vi "Nimbelink_Database_Ops.vi"(0 "Operation":T1(ring)=enum."Get Col Names", 1 "Record data":string[](array[string])=["wo12345", "123450001", "70B3D55A8100", "A1001234567890", "Joe", "2013-05-07 10:28:19", "100013", "353123456789012", "89123456789012345678", "612-555-1212", "Pass", "", "", "", "", "", "", "", "", "", "", "", "", "", "", "", "", "", "", "", "", "", "", "", "", "", "", "", "", "", "", "", "", "", "", "", "", "", "", "", "", "", "", "", "", "", "", "", "", "", "", "", "12:01:00"], 2 "Open SQL session?":bool=TRUE, 3 "Connection In":refnum<k7>, 4 "SQL Query":string="Insert into dbo.test_data VALUES ", 5 "Error in (no error)":errorcluster, 6 "Find column":u16(ring) items=["work_order", "btw_sn", "mac", "meid", "operator", "datetime", "part_number", "imei", "sim_id", "phone", "test_result"], 7 "Find data":string, 10 "table name":string="test_data", 11 "Insert fields":i32=23) -> (12 "Found?":bool, 13 "Last test passed?":bool, 14 "RecordSet":string[][](array[string]), 15 "Column Names":string[](array[string])=["work_order", "btw_sn", "mac", "meid", "operator", "date_time", "part_number", "imei", "sim_id", "phone_number", "test_result", "board_sn", "test_time", "test_program", "test_version", "extra1", "extra2", "guid", "extra3", "extra4", "extra5", "extra6", "extra7"], 16 "Connection Out":refnum<k7>, 17 "Find return string":string, 18 "Records":i32, 19 "Error out":errorcluster)   [LabVIEW 2013]
panel:
  out "Final query string":string="select column_name,* from information_schema.columns\n where table_name = 'test_data'\norder by ordinal_position"
  in  "ConnectionString":string="Provider=SQLOLEDB.1;User Id=SSTest;Password=test;Initial Catalog=Nimbelink;Data Source=BTWSQLSVR\\TESTDEPT "
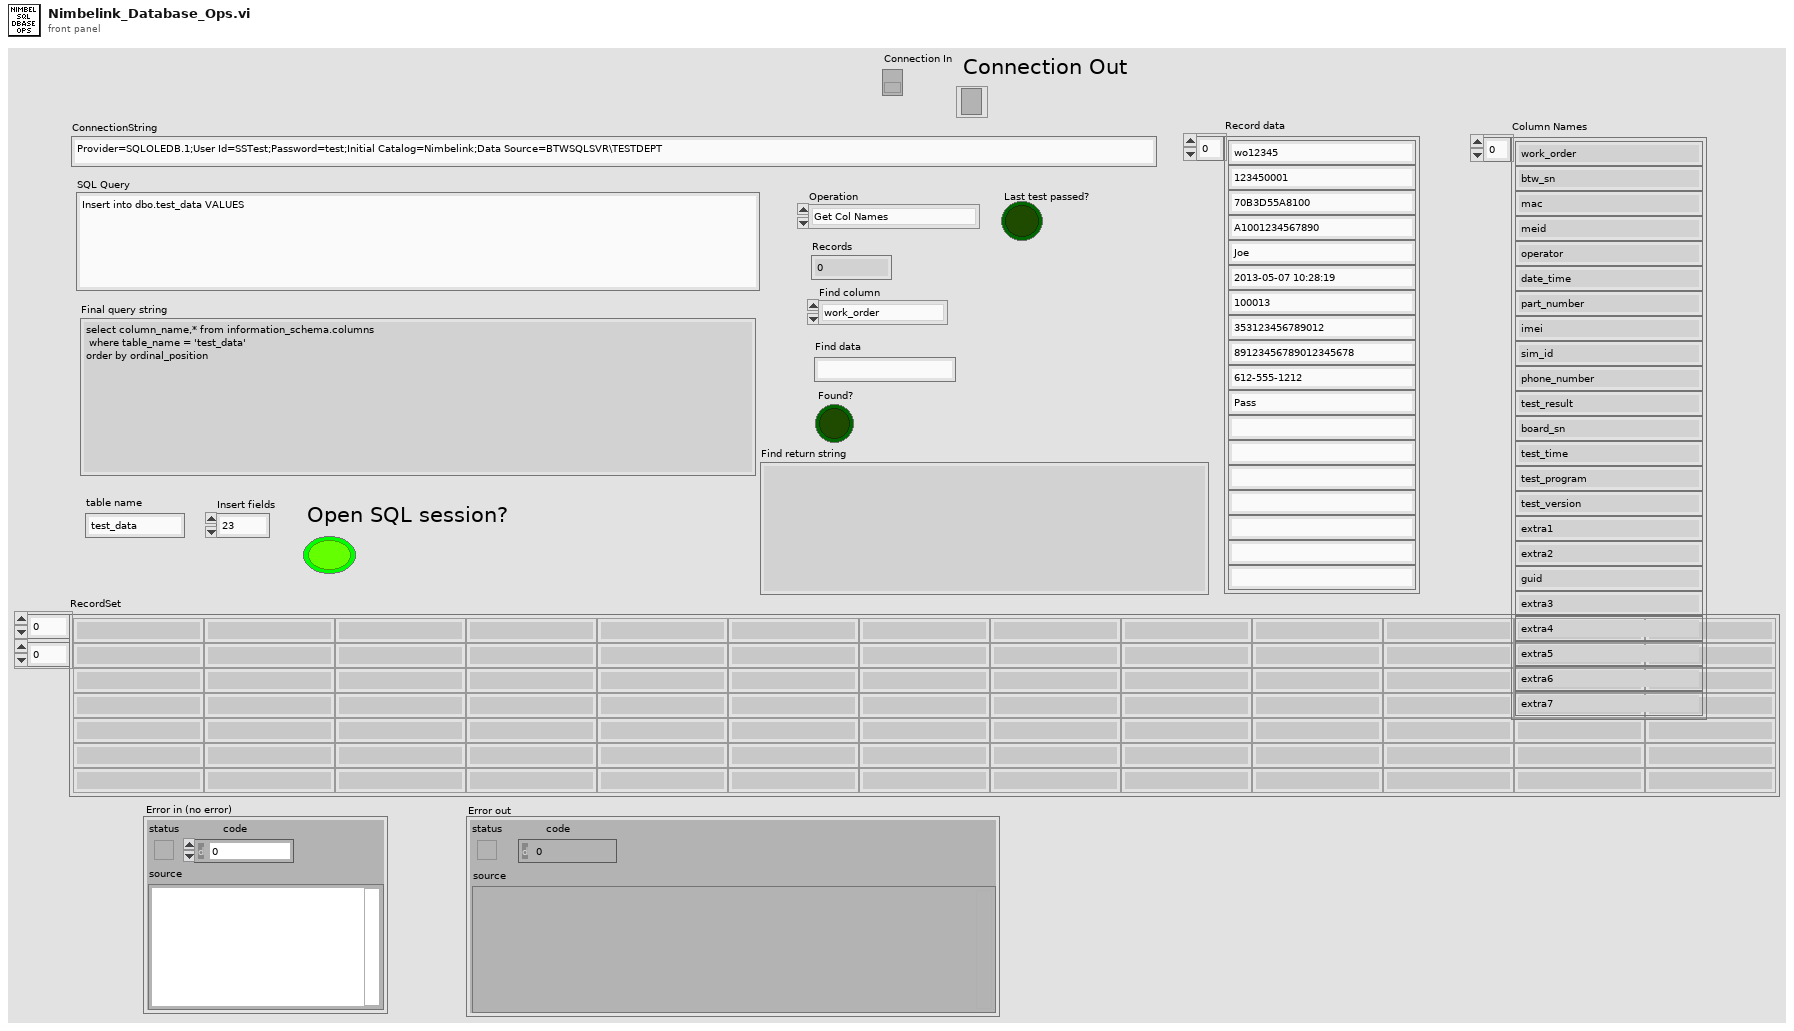
[diagram p1: front panel]
types:
  T1 = enum16{"Query", "Insert", "Select", "Dump Recs", "Get Rec Count", "Get Col Names", "Insert all fields", "Find", "Get last test result", "Get work order qty", "Set work order qty", "Save test report", "Get test report", "Execute query no data", "Select count", "Query and return row 0 col 0"}
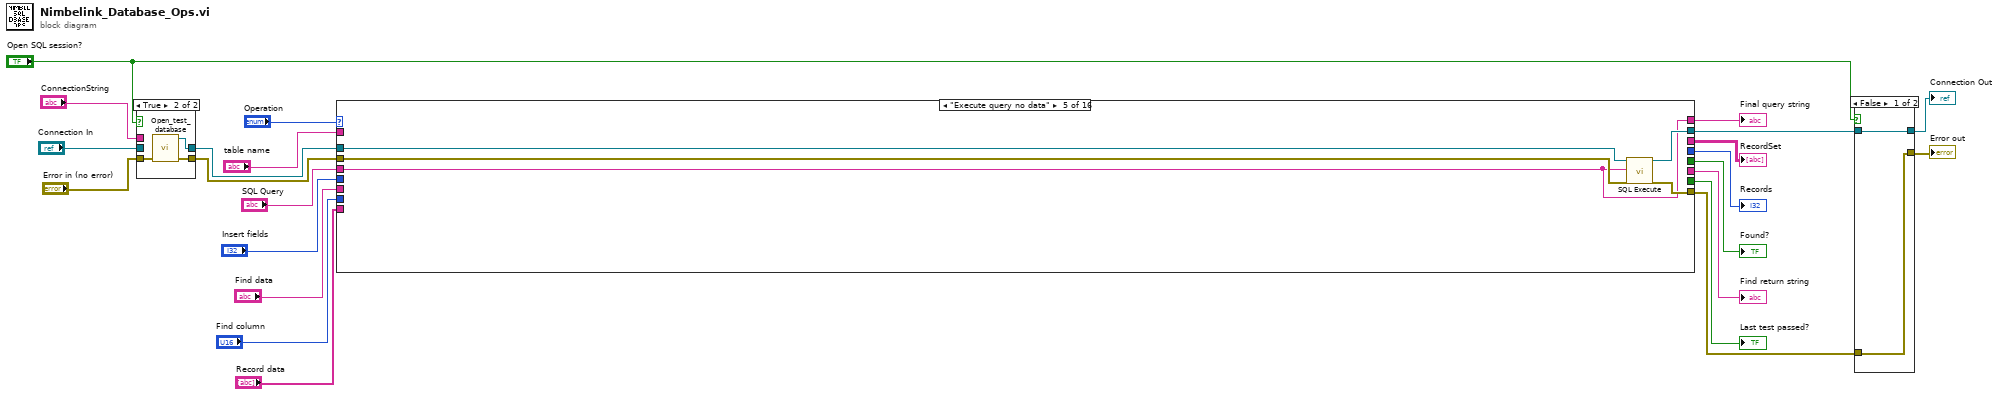
[diagram p0: block diagram]
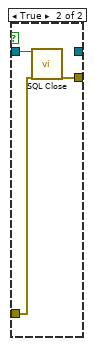
[diagram p2: hidden frame]
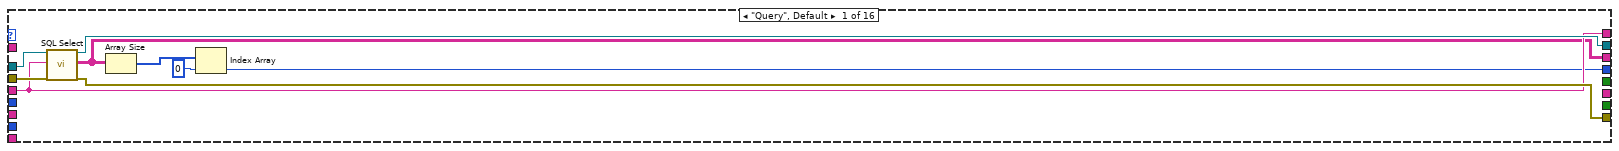
[diagram p4: hidden frame]
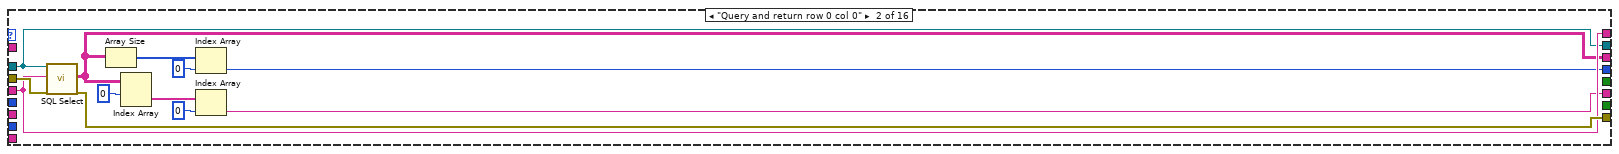
[diagram p5: hidden frame]
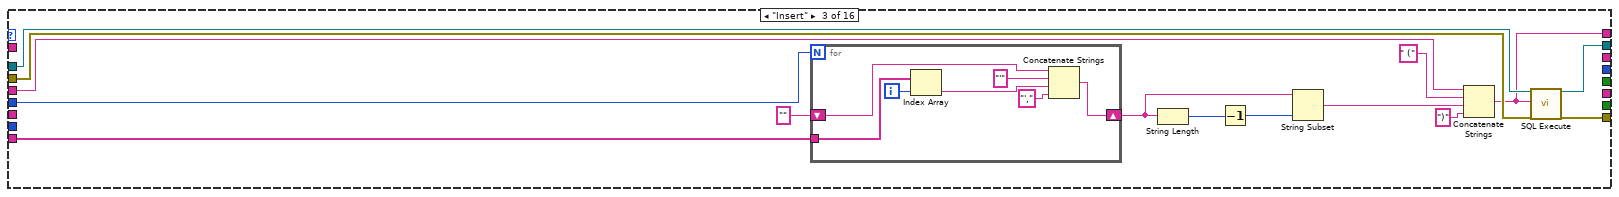
[diagram p6: hidden frame]
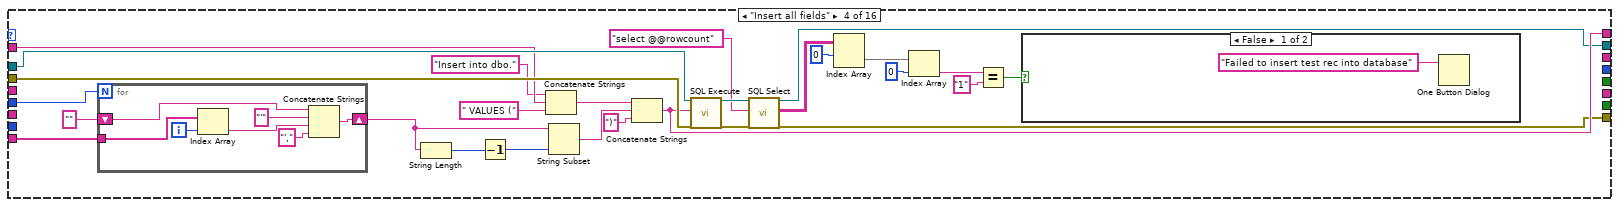
[diagram p7: hidden frame]
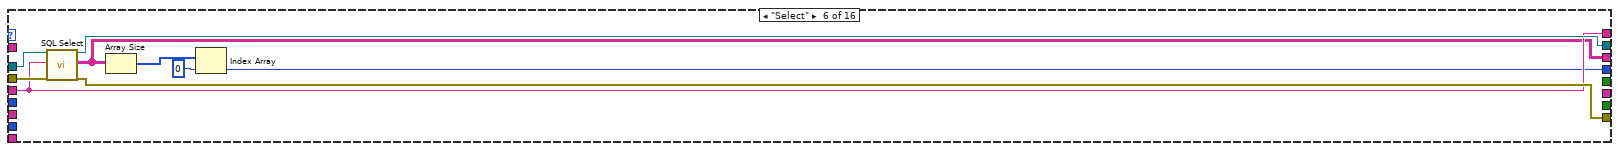
[diagram p9: hidden frame]
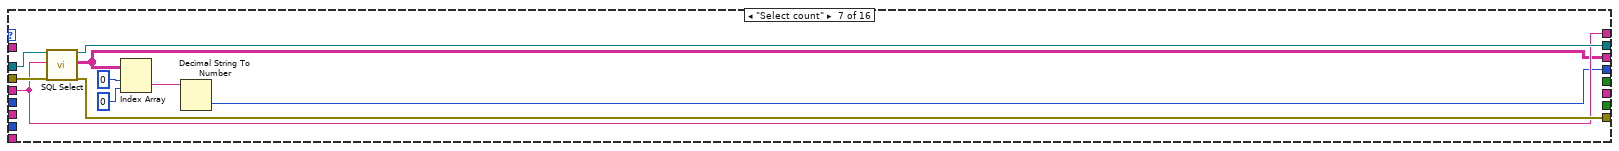
[diagram p10: hidden frame]
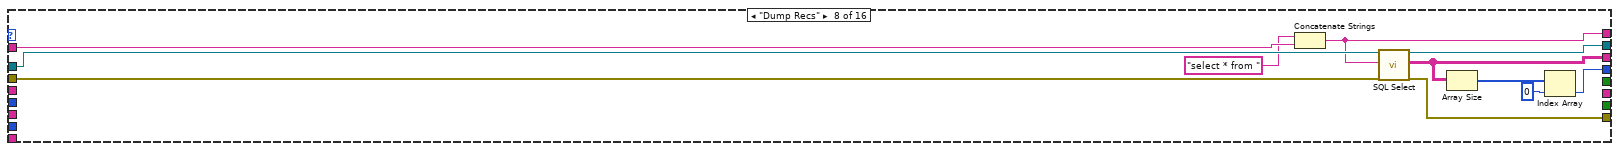
[diagram p11: hidden frame]
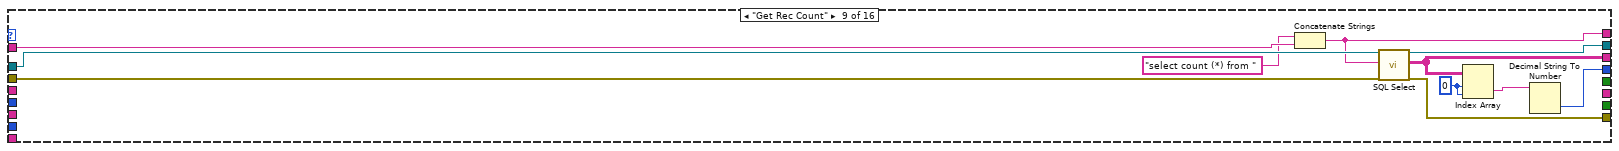
[diagram p12: hidden frame]
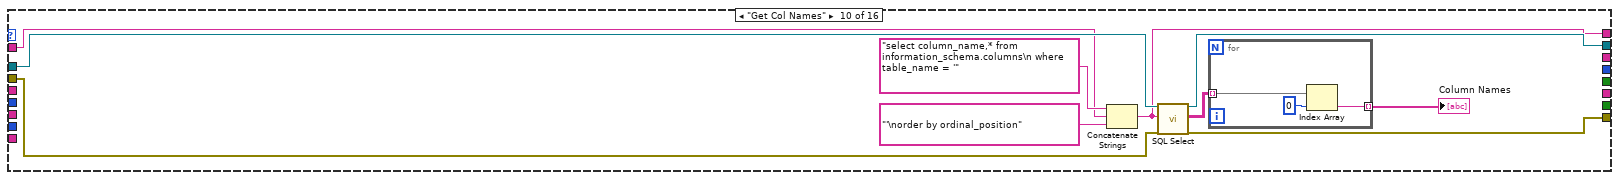
[diagram p13: hidden frame]
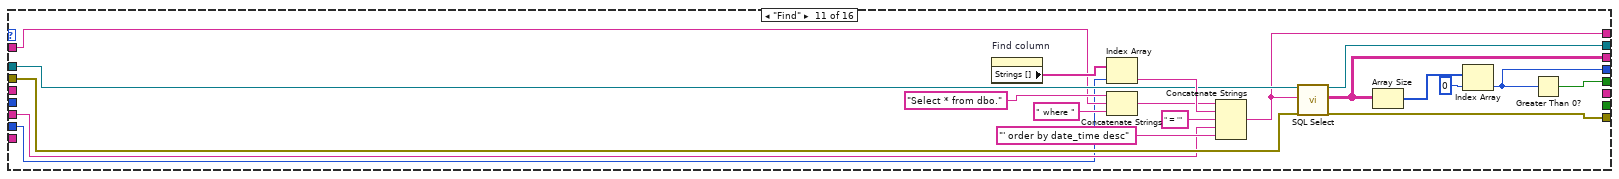
[diagram p14: hidden frame]
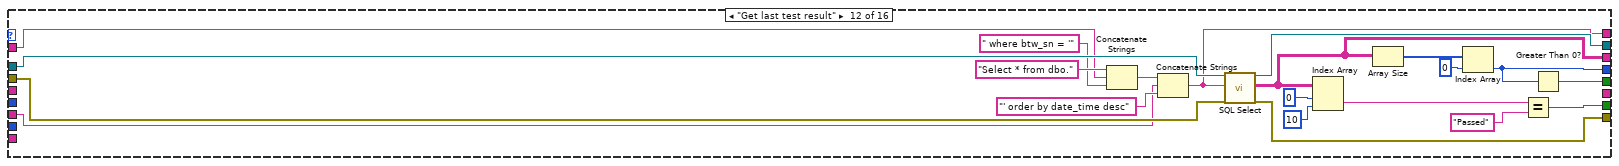
[diagram p15: hidden frame]
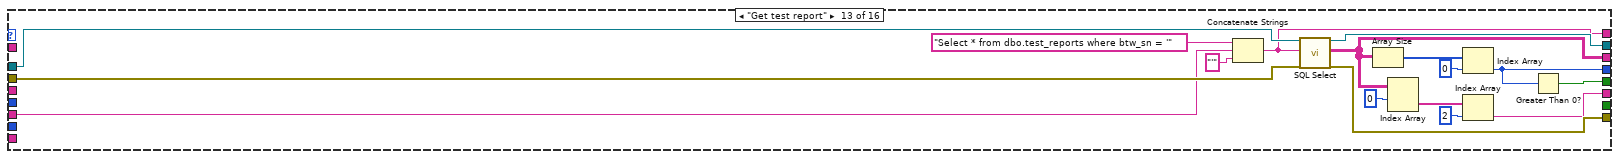
[diagram p16: hidden frame]
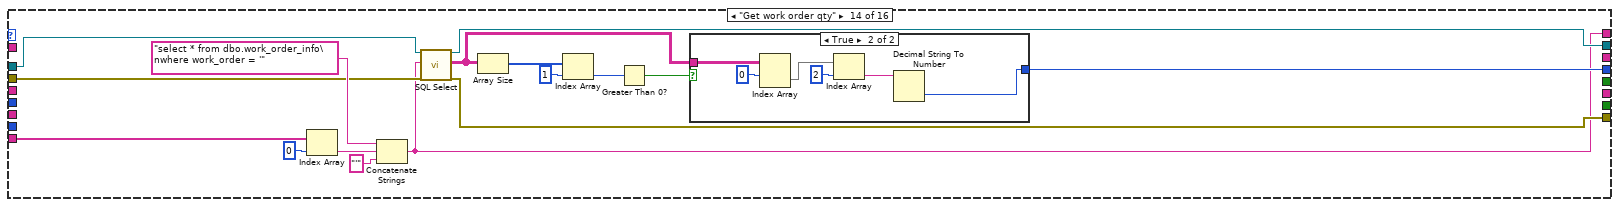
[diagram p17: hidden frame]
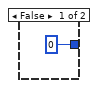
[diagram p18: hidden frame]
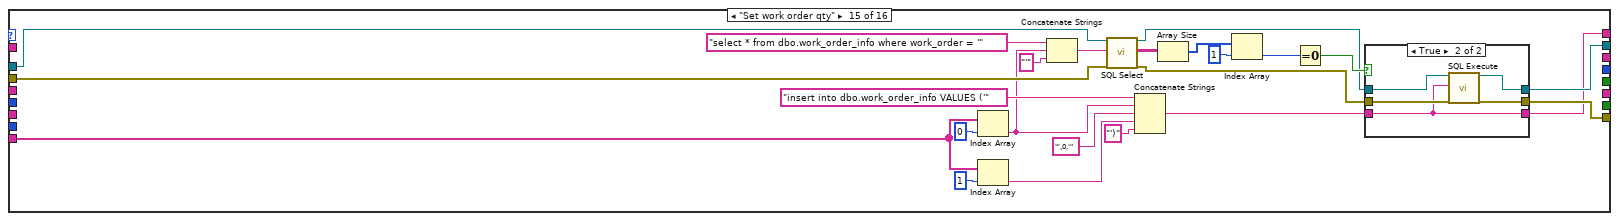
[diagram p19: hidden frame]
diagram:
  n1 = case shown="True" "Open SQL session?" {
    tunnel: "ConnectionString" -> [_ _]
    tunnel: "Error in (no error)" -> [w24 w28]
    tunnel: [w25 w26] -> w19
    tunnel: [w24 w27] -> w18
    tunnel: "Connection In" -> [w25 _]
    frame False {
    }
    frame True {
      n2 = call "Open_test_database.vi"("error in (no error)"=w28) -> ("error out"=w27:errorcluster, "SQL conn Refnum out"=w26:refnum<k7>)  [unwired: 9 in]
    }
  }
  n3 = case shown="\"Execute query no data\"" "Operation" {
    tunnel: [w36 w48 w64 w73 w111 w117 w127 w138 w149 w158 w179 w203 w220 w228 w254 w288] -> w21
    tunnel: [w34 w38 w63 w72 w110 w118 w128 w139 w150 w157 w181 w205 w222 w230 w253 w287] -> w20
    tunnel: w19 -> [w35 w38 w62 w98 w109 w119 w129 w141 w152 w162 w182 w206 w223 w231 w270 w284]
    tunnel: w18 -> [w37 w49 w52 w90 w108 w120 w130 w140 w151 w161 w180 w204 w221 w233 w267 w285]
    tunnel: "SQL Query" -> [w33 w47 w57 _ w107 w116 w126 _ _ _ _ _ _ _ _ _]
    tunnel: [w30 w43 _ _ _ w113 w124 w134 w144 _ w176 w191 w211 _ _ _] -> w1
    tunnel: "Record data" -> [_ _ w61 w97 _ _ _ _ _ _ _ _ _ w232 w259 w283]
    tunnel: [w33 w47 w51 w89 w107 w116 w126 w137 w146 w156 w175 w200 w217 w227 w252 w286] -> w13
    tunnel: "table name" -> [_ _ _ w88 _ _ _ w136 w147 w154 w172 w197 _ _ _ _]
    tunnel: [w29 w44 _ _ _ w112 w123 w131 w143 _ w169 w194 w215 w229 _ _] -> w11
    tunnel: [_ _ _ _ _ _ _ _ _ _ w168 w193 w214 _ _ _] -> w10
    tunnel: "Find data" -> [_ _ _ _ _ _ _ _ _ _ w167 w192 w213 _ _ _]
    tunnel: "Find column" -> [_ _ _ _ _ _ _ _ _ _ w166 _ _ _ _ _]
    tunnel: [_ _ _ _ _ _ _ _ _ _ _ w186 _ _ _ _] -> w7
    tunnel: "Insert fields" -> [_ _ w50 w84 _ _ _ _ _ _ _ _ _ _ _ _]
    tunnel: [_ w39 _ _ _ _ _ _ _ _ _ _ w208 _ _ _] -> w5
    frame "Query", Default {
      n4 = call "SQL Select.vi"("Connection In"=w35, "SQL Query"=w33, "Error in (no error)"=w37) -> ("Connection Out"=w34:refnum<k7>, "Data"=w30:string[][], "Error out"=w36:errorcluster)  [unwired: 14 in]
      n5 = Array Size(array=w30) -> (size(s)=w32:i32[])
      n6 = Index Array(array=w32, index=0) -> (element=w29:i32)
    }
    frame "Query and return row 0 col 0" {
      n7 = call "SQL Select.vi"("Connection In"=w38, "SQL Query"=w47, "Error in (no error)"=w49) -> ("Data"=w43:string[][], "Error out"=w48:errorcluster)  [unwired: 14 in, 1 out]
      n8 = Array Size(array=w43) -> (size(s)=w46:i32[])
      n9 = Index Array(array=w43, index (row)=0) -> (element=w41:string[])  [unwired: 1 in]
      n10 = Index Array(array=w46, index=0) -> (element=w44:i32)
      n11 = Index Array(array=w41, index=0) -> (element=w39:string)
    }
    frame "Insert" {
      n12 = for {
        N: w50 -> [_]
        tunnel: w61 -> [w67]
        shift-right: [w70] -> w54
        shift-left: "" -> [w69]
        i -> [w66]
        n13 = Index Array(array=w67, index=w66) -> (element=w65:string)
        n14 = Concatenate Strings(w69, "'" ("string"), w65, "'," ("string")) -> (w70:string)
      }
      n15 = String Length(string=w54) -> (length=w56:i32)
      n16 = Decrement(x=w56) -> (x-1=w55:i32)
      n17 = String Subset(string=w54, length (rest)=w55) -> (substring=w53:string)  [unwired: 1 in]
      n18 = Concatenate Strings(w57, " (" ("string"), w53, ")") -> (w51:string)
      n19 = call "SQL Execute.vi"("Connection In"=w62, "SQL Query"=w51, "Error in (no error)"=w52) -> ("Connection Out"=w63:refnum<k7>, "Error out"=w64:errorcluster)  [unwired: 15 in]
    }
    frame "Insert all fields" {
      n20 = for {
        N: w84 -> [_]
        tunnel: w97 -> [w102]
        shift-right: [w105] -> w92
        shift-left: "" -> [w104]
        i -> [w101]
        n21 = Index Array(array=w102, index=w101) -> (element=w100:string)
        n22 = Concatenate Strings(w104, "'" ("string"), w100, "'," ("string")) -> (w105:string)
      }
      n23 = String Length(string=w92) -> (length=w94:i32)
      n24 = Decrement(x=w94) -> (x-1=w93:i32)
      n25 = Concatenate Strings("Insert into dbo." ("string"), w88, " VALUES (" ("string")) -> (w87:string)
      n26 = String Subset(string=w92, length (rest)=w93) -> (substring=w91:string)  [unwired: 1 in]
      n27 = Concatenate Strings(w87, w91, ")") -> (w89:string)
      n28 = call "SQL Execute.vi"("Connection In"=w98, "SQL Query"=w89, "Error in (no error)"=w90) -> ("Connection Out"=w83:refnum<k7>, "Error out"=w82:errorcluster)  [unwired: 15 in]
      n29 = call "SQL Select.vi"("Connection In"=w83, "SQL Query"="select @@rowcount", "Error in (no error)"=w82) -> ("Connection Out"=w72:refnum<k7>, "Data"=w80:string[][], "Error out"=w73:errorcluster)  [unwired: 14 in]
      n30 = Index Array(array=w80, index (row)=0) -> (element=w78:string[])  [unwired: 1 in]
      n31 = Index Array(array=w78, index=0) -> (element=w76:string)
      n32 = Equal?(x=w76, y="1") -> (x = y?=w74:bool)
      n33 = case shown="False" w74 {
        frame False {
          n34 = One Button Dialog(message="Failed to insert test rec into database" ("string")) -> ()  [unwired: 1 in, 1 out]
        }
        frame True {
        }
      }
    }
    frame "Execute query no data" {
      n35 = call "SQL Execute.vi"("Connection In"=w109, "SQL Query"=w107, "Error in (no error)"=w108) -> ("Connection Out"=w110:refnum<k7>, "Error out"=w111:errorcluster)  [unwired: 15 in]
    }
    frame "Select" {
      n36 = call "SQL Select.vi"("Connection In"=w119, "SQL Query"=w116, "Error in (no error)"=w120) -> ("Connection Out"=w118:refnum<k7>, "Data"=w113:string[][], "Error out"=w117:errorcluster)  [unwired: 14 in]
      n37 = Array Size(array=w113) -> (size(s)=w115:i32[])
      n38 = Index Array(array=w115, index=0) -> (element=w112:i32)
    }
    frame "Select count" {
      n39 = call "SQL Select.vi"("Connection In"=w129, "SQL Query"=w126, "Error in (no error)"=w130) -> ("Connection Out"=w128:refnum<k7>, "Data"=w124:string[][], "Error out"=w127:errorcluster)  [unwired: 14 in]
      n40 = Index Array(array=w124, index (row)=0, index (col)=0 ("disabled index (col)")) -> (element=w121:string)
      n41 = Decimal String To Number(string=w121) -> (number=w123:i32)  [unwired: 2 in, 1 out]
    }
    frame "Dump Recs" {
      n42 = Concatenate Strings("select * from " ("SQL Query"), w136) -> (w137:string)
      n43 = call "SQL Select.vi"("Connection In"=w141, "SQL Query"=w137, "Error in (no error)"=w140) -> ("Connection Out"=w139:refnum<k7>, "Data"=w134:string[][], "Error out"=w138:errorcluster)  [unwired: 14 in]
      n44 = Array Size(array=w134) -> (size(s)=w133:i32[])
      n45 = Index Array(array=w133, index=0) -> (element=w131:i32)
    }
    frame "Get Rec Count" {
      w148 = 0 ("index (row)")
      n46 = Concatenate Strings("select count (*) from " ("SQL Query"), w147) -> (w146:string)
      n47 = call "SQL Select.vi"("Connection In"=w152, "SQL Query"=w146, "Error in (no error)"=w151) -> ("Connection Out"=w150:refnum<k7>, "Data"=w144:string[][], "Error out"=w149:errorcluster)  [unwired: 14 in]
      n48 = Index Array(array=w144, index (row)=w148, index (col)=w148) -> (element=w142:string)
      n49 = Decimal String To Number(string=w142) -> (number=w143:i32)  [unwired: 2 in, 1 out]
    }
    frame "Get Col Names" {
      n50 = Concatenate Strings("select column_name,* from information_schema.columns\n where table_name = '" ("SQL Query"), w154, "'\norder by ordinal_position" ("SQL Query")) -> (w156:string)
      n51 = call "SQL Select.vi"("Connection In"=w162, "SQL Query"=w156, "Error in (no error)"=w161) -> ("Connection Out"=w157:refnum<k7>, "Data"=w160:string[][], "Error out"=w158:errorcluster)  [unwired: 14 in]
      n52 = for {
        tunnel: w160 -> [w165] mode=indexing
        tunnel: [w164] -> w159 mode=indexing
        n53 = Index Array(array=w165, index=0 ("index (col)")) -> (element=w164:string)
      }
      "Column Names" <- w159
    }
    frame "Find" {
      n54 = property on="Find column" class="Ring (strict)"() -> ("Strings []"=w185:string[])  [unwired: 2 in, 2 out]
      n55 = Index Array(array=w185, index=w166) -> (element=w184:string)
      n56 = Concatenate Strings("Select * from dbo." ("string"), w172, " where " ("string")) -> (w174:string)
      n57 = Concatenate Strings(w174, w184, " = '" ("string"), w167, "' order by date_time desc" ("string")) -> (w175:string)
      n58 = call "SQL Select.vi"("Connection In"=w182, "SQL Query"=w175, "Error in (no error)"=w180) -> ("Connection Out"=w181:refnum<k7>, "Data"=w176:string[][], "Error out"=w179:errorcluster)  [unwired: 14 in]
      n59 = Array Size(array=w176) -> (size(s)=w177:i32[])
      n60 = Index Array(array=w177, index=0) -> (element=w169:i32)
      n61 = Greater Than 0?(x=w169) -> (x > 0?=w168:bool)
    }
    frame "Get last test result" {
      n62 = Concatenate Strings("Select * from dbo." ("string"), w197, " where btw_sn = '" ("string")) -> (w199:string)
      n63 = Concatenate Strings(w199, w192, "' order by date_time desc" ("string")) -> (w200:string)
      n64 = call "SQL Select.vi"("Connection In"=w206, "SQL Query"=w200, "Error in (no error)"=w204) -> ("Connection Out"=w205:refnum<k7>, "Data"=w191:string[][], "Error out"=w203:errorcluster)  [unwired: 14 in]
      n65 = Index Array(array=w191, index (row)=0, index (col)=10 ("disabled index (col)")) -> (element=w188:string)
      n66 = Array Size(array=w191) -> (size(s)=w201:i32[])
      n67 = Index Array(array=w201, index=0) -> (element=w194:i32)
      n68 = Equal?(x=w188, y="Passed") -> (x = y?=w186:bool)
      n69 = Greater Than 0?(x=w194) -> (x > 0?=w193:bool)
    }
    frame "Get test report" {
      n70 = Concatenate Strings("Select * from dbo.test_reports where btw_sn = '" ("string"), w213, "'" ("string")) -> (w217:string)
      n71 = call "SQL Select.vi"("Connection In"=w223, "SQL Query"=w217, "Error in (no error)"=w221) -> ("Connection Out"=w222:refnum<k7>, "Data"=w211:string[][], "Error out"=w220:errorcluster)  [unwired: 14 in]
      n72 = Array Size(array=w211) -> (size(s)=w218:i32[])
      n73 = Index Array(array=w211, index (row)=0) -> (element=w209:string[])  [unwired: 1 in]
      n74 = Index Array(array=w218, index=0) -> (element=w215:i32)
      n75 = Index Array(array=w209, index=2) -> (element=w208:string)
      n76 = Greater Than 0?(x=w215) -> (x > 0?=w214:bool)
    }
    frame "Get work order qty" {
      n77 = Index Array(array=w232, index=0) -> (element=w235:string)
      n78 = Concatenate Strings("select * from dbo.work_order_info\nwhere work_order = '" ("SQL Query"), w235, "'" ("string")) -> (w227:string)
      n79 = call "SQL Select.vi"("Connection In"=w231, "SQL Query"=w227, "Error in (no error)"=w233) -> ("Connection Out"=w230:refnum<k7>, "Data"=w226:string[][], "Error out"=w228:errorcluster)  [unwired: 14 in]
      n80 = Array Size(array=w226) -> (size(s)=w225:i32[])
      n81 = Index Array(array=w225, index=1) -> (element=w224:i32)
      n82 = Greater Than 0?(x=w224) -> (x > 0?=w234:bool)
      n83 = case shown="True" w234 {
        tunnel: w226 -> [_ w245]
        tunnel: [0 w244] -> w229
        frame False {
        }
        frame True {
          n84 = Index Array(array=w245, index (row)=0 ("index")) -> (element=w243:string[])  [unwired: 1 in]
          n85 = Index Array(array=w243, index=2) -> (element=w241:string)
          n86 = Decimal String To Number(string=w241) -> (number=w244:i32)  [unwired: 2 in, 1 out]
        }
      }
    }
    frame "Set work order qty" {
      n87 = Index Array(array=w259, index=0) -> (element=w258:string)
      n88 = Index Array(array=w259, index=1) -> (element=w260:string)
      n89 = Concatenate Strings("select * from dbo.work_order_info where work_order = '" ("SQL Query"), w258, "'" ("string")) -> (w251:string)
      n90 = call "SQL Select.vi"("Connection In"=w270, "SQL Query"=w251, "Error in (no error)"=w267) -> ("Connection Out"=w256:refnum<k7>, "Data"=w247:string[][], "Error out"=w255:errorcluster)  [unwired: 14 in]
      n91 = Concatenate Strings("insert into dbo.work_order_info VALUES ('" ("SQL Query"), w258, "',0,'" ("string"), w260, "')" ("string")) -> (w248:string)
      n92 = Array Size(array=w247) -> (size(s)=w250:i32[])
      n93 = Index Array(array=w250, index=1) -> (element=w249:i32)
      n94 = Equal To 0?(x=w249) -> (x = 0?=w265:bool)
      n95 = case shown="True" w265 {
        tunnel: w256 -> [w272 w275]
        tunnel: w248 -> [w271 w274]
        tunnel: w255 -> [w273 w278]
        tunnel: [w273 w277] -> w254
        tunnel: [w272 w276] -> w253
        tunnel: [w271 w274] -> w252
        frame False {
        }
        frame True {
          n96 = call "SQL Execute.vi"("Connection In"=w275, "SQL Query"=w274, "Error in (no error)"=w278) -> ("Connection Out"=w276:refnum<k7>, "Error out"=w277:errorcluster)  [unwired: 15 in]
        }
      }
    }
    frame "Save test report" {
      w281 = "','" ("string")
      n97 = Index Array(array=w283, index=0) -> (element=w289:string)
      n98 = Index Array(array=w283, index=1) -> (element=w290:string)
      n99 = Index Array(array=w283, index=2) -> (element=w280:string)
      n100 = Concatenate Strings("insert into dbo.test_reports values ('" ("SQL Query"), w289, w281, w290, w281, w280, "')" ("string")) -> (w286:string)
      n101 = call "SQL Execute.vi"("Connection In"=w284, "SQL Query"=w286, "Error in (no error)"=w285) -> ("Connection Out"=w287:refnum<k7>, "Error out"=w288:errorcluster)  [unwired: 15 in]
    }
  }
  "RecordSet" <- w1
  "Final query string" <- w13
  "Records" <- w11
  "Found?" <- w10
  "Last test passed?" <- w7
  "Find return string" <- w5
  n102 = case shown="False" "Open SQL session?" {
    tunnel: w21 -> [w295 w298]
    tunnel: w20 -> [w294 w297]
    tunnel: [w295 w296] -> w17
    tunnel: [w294 _] -> w2
    frame False {
    }
    frame True {
      n103 = call "SQL Close.vi"("Connection In"=w297, "Error in (no error)"=w298) -> ("Error out"=w296:errorcluster)  [unwired: 17 in]
    }
  }
  "Error out" <- w17
  "Connection Out" <- w2
